vi "login.vi"() -> (3 "client handle out":T1)   [LabVIEW 2012]
uses:
  Key-Value Pair.ctl
  <vilib>/httpClient/ClientHandle.ctl
  <vilib>/httpClient/POSTBuffer.vi
  <vilib>/httpClient/LabVIEWHTTPClient.lvlib
panel:
  out "response code from final location":i32
  out "Parsed Headers":T2[](array[typedef])
  out "Value":string
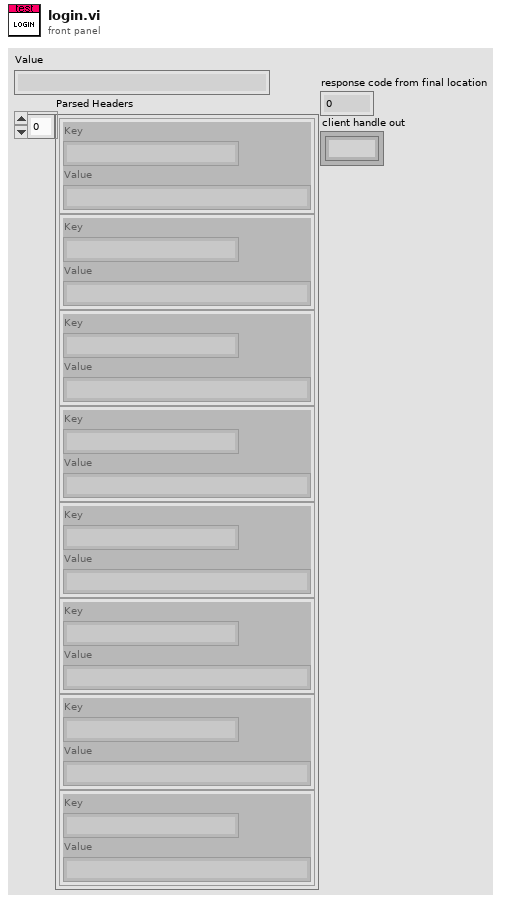
[diagram p1: front panel]
types:
  T1 = typedef "LabVIEWHTTPClient.lvlib/ClientHandle.ctl" = refnum<k1>
  T2 = typedef "Key-Value Pair.ctl" = cluster{"Key":string, "Value":string}
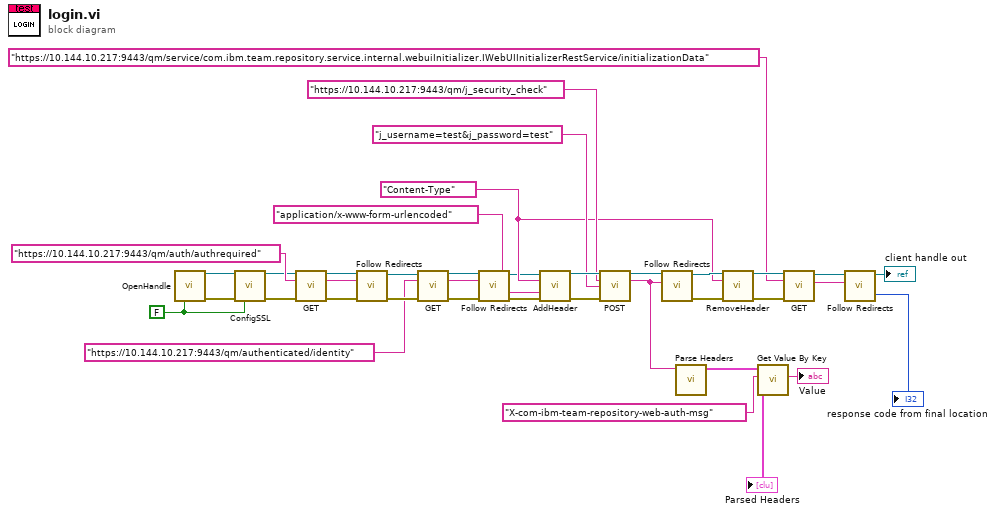
[diagram p0: block diagram]
diagram:
  w22 = "Content-Type" ("header")
  w26 = FALSE ("verify server(true)")
  n1 = call <vilib>:"OpenHandle.vi"("verify server(true)"=w26) -> ("client handle out"=w37:T1, "error out"=w36:errorcluster)  [unwired: 13 in]
  n2 = call <vilib>:"ConfigSSL.vi"("client handle"=w37, "error in (no error)"=w36, "verify server (true)"=w26) -> ("client handle out"=w25:T1, "error out"=w35:errorcluster)  [unwired: 11 in]
  n3 = call <vilib>:"GET.vi"("client handle"=w25, "url"="https://10.144.10.217:9443/qm/auth/authrequired", "error in (no error)"=w35) -> ("client handle out"=w10:T1, "headers"=w8:string, "error out"=w7:errorcluster)  [unwired: 9 in, 1 out]
  n4 = call "Follow Redirects.vi"("error in (no error)"=w7, "Headers"=w8, "client handle"=w10) -> ("error out"=w6:errorcluster, "client handle out"=w9:T1)  [unwired: 4 in, 3 out]
  n5 = call <vilib>:"GET.vi"("client handle"=w9, "url"="https://10.144.10.217:9443/qm/authenticated/identity", "error in (no error)"=w6) -> ("client handle out"=w4:T1, "headers"=w3:string, "error out"=w5:errorcluster)  [unwired: 9 in, 1 out]
  n6 = call "Follow Redirects.vi"("error in (no error)"=w5, "Headers"=w3, "client handle"=w4) -> ("error out"=w11:errorcluster, "client handle out"=w12:T1)  [unwired: 4 in, 3 out]
  n7 = call <vilib>:"AddHeader.vi"("client handle"=w12, "header"=w22, "value"="application/x-www-form-urlencoded", "error in (no error)"=w11) -> ("client handle out"=w32:T1, "error out"=w29:errorcluster)  [unwired: 10 in]
  n8 = call-poly <vilib>:"POST.vi"("client handle"=w32, "url"="https://10.144.10.217:9443/qm/j_security_check", "buffer"="j_username=test&j_password=test", "error in (no error)"=w29) -> ("client handle out"=w20:T1, "headers"=w24:string)  [unwired: 8 in, 2 out]
  n9 = call "Follow Redirects.vi"("Headers"=w24, "client handle"=w20) -> ("error out"=w21:errorcluster, "client handle out"=w23:T1)  [unwired: 5 in, 3 out]
  n10 = call "Parse Headers.vi"("Raw Header"=w24) -> ("Parsed Headers"=w28:T2[])  [unwired: 9 in, 1 out]
  "Parsed Headers" <- w28
  n11 = call <vilib>:"RemoveHeader.vi"("client handle"=w23, "header"=w22, "error in (no error)"=w21) -> ("client handle out"=w18:T1, "error out"=w16:errorcluster)  [unwired: 11 in]
  n12 = call "Get Value By Key.vi"("Key"="X-com-ibm-team-repository-web-auth-msg", "Key-Value Pairs"=w28) -> ("Value"=→"Value":string)  [unwired: 9 in]
  n13 = call <vilib>:"GET.vi"("client handle"=w18, "url"="https://10.144.10.217:9443/qm/service/com.ibm.team.repository.service.internal.webuiInitializer.IWebUIInitializerRestService/initializationData", "error in (no error)"=w16) -> ("client handle out"=w15:T1, "headers"=w14:string)  [unwired: 9 in, 2 out]
  n14 = call "Follow Redirects.vi"("Headers"=w14, "client handle"=w15) -> ("client handle out"=→"client handle out":T1, "response code from final location"=→"response code from final location":i32)  [unwired: 5 in, 3 out]
